vi "PLC_Main.vi"() -> ()   [LabVIEW 2017]
doc: "Andon System cards scanning and ouput ON/OFF through MQTT protocol. Update data in SQL data base for reporting."
uses:
  Control/Andon_demo State.ctl
  <vilib>/addons/database/NI_Database_API.lvlib
  <vilib>/NI/Modbus Library/API/Wrapper/API Main.lvlib
  <vilib>/NI/Modbus Library/API/Wrapper/Create TCP Master.vi
  <vilib>/NI/Modbus Library/API/master/Modbus Master.lvclass
  <vilib>/addons/database/Connection.llb/DB Tools Open Connec (Path).vi
  <vilib>/addons/database/Connection.llb/Conn ObjectReference.ctl
panel:
  out "PLC Status":bool[](array[boolean])
  out "Modbus Instances":refnum<class "Modbus Master.lvclass">[](array[class])
  out "State to Log":T1(array[cluster])
  out "Input Status":bool[][](array[boolean])
  out "Output Status":bool[][](array[boolean])
  in  "stop":bool
  out "Stop from Main":bool
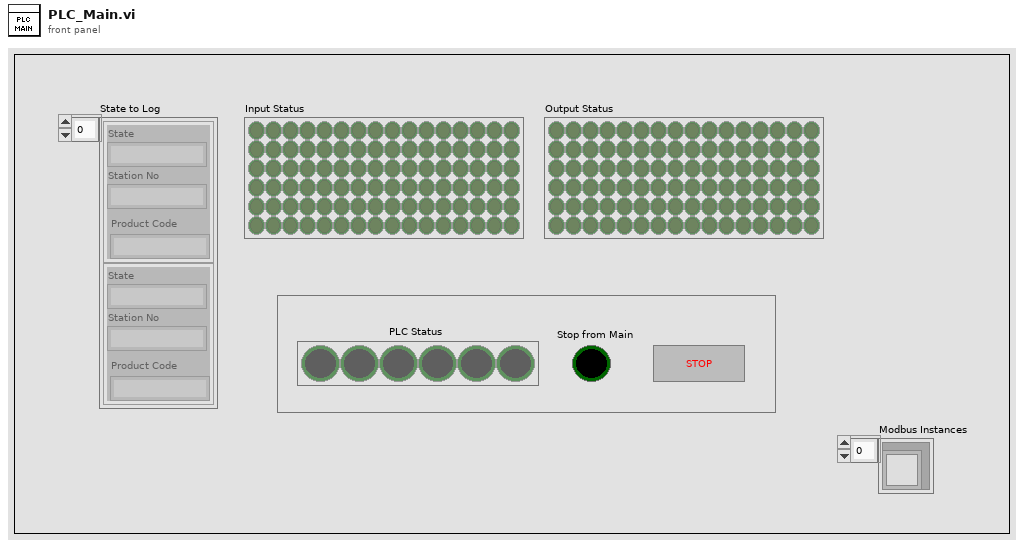
[diagram p1: front panel]
types:
  T1 = cluster{"State":string, "Station No":string, "Product Code":string}[]
  T2 = enum32{"Invalid", "Standard", "Closed", "Hidden", "Minimized", "Maximized"}
  T3 = cluster{"State":string, "Station No":string, "Product Code":string}
  T4 = typedef "Andon_demo State.ctl" = enum16{"Initialise", "Read Inputs", "Process Inputs", "Generate Log Trigger"}
  T5 = cluster{"TCP master instance":refnum<class "Modbus Master.lvclass">, "error out":errorcluster, "CID":string}[]
  T6 = cluster{"TCP master instance":refnum<class "Modbus Master.lvclass">, "error out":errorcluster, "CID":string}
  T7 = cluster{"CID":string, "Comm Stat":bool, "Input":u16[]}
  T8 = typedef "NI_Database_API.lvlib/Conn ObjectReference.ctl" = refnum<k1>
  T9 = cluster{"client name":string, "broker/ server ip address":string[]}
  T10 = cluster{"CID":string, "Comm Stat":bool, "Input":u16[]}[]
  T11 = enum32{"invalid app kind", "Development System", "Run Time System", "Student Edition", "Embedded LabVIEW", "Evaluation", "Custom"}
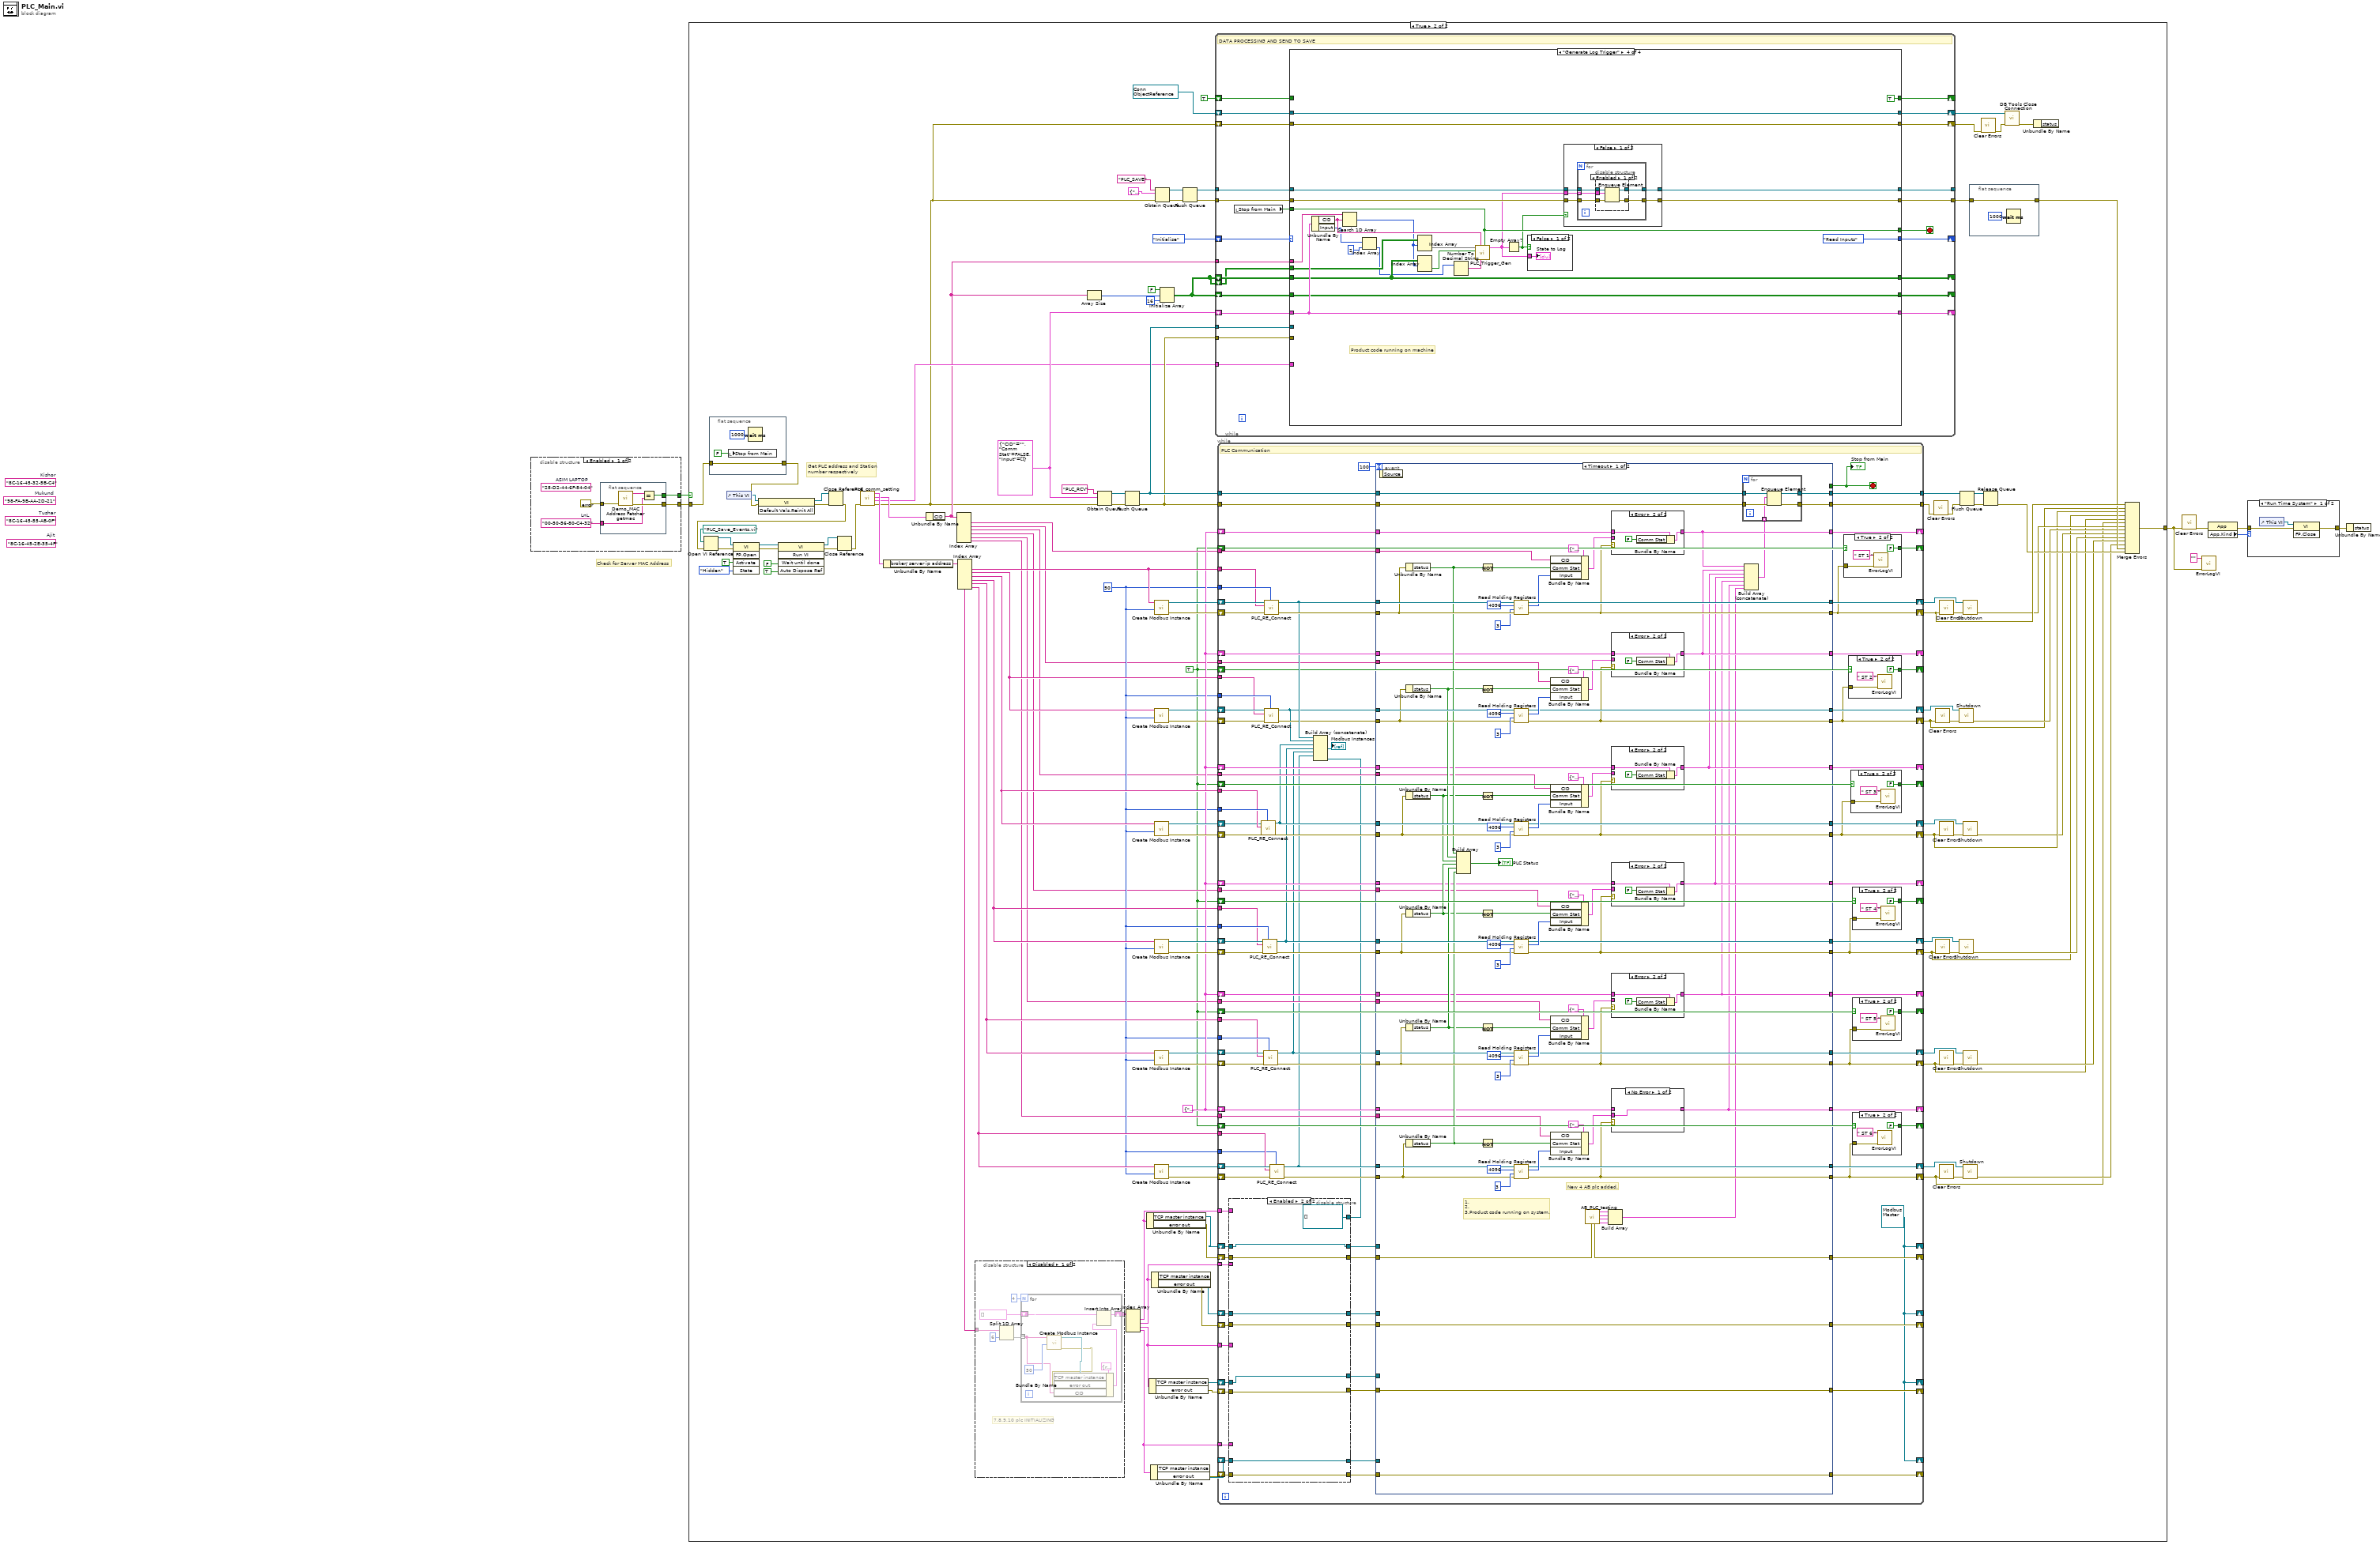
[diagram p0: block diagram]
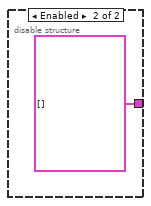
[diagram p3: hidden frame]
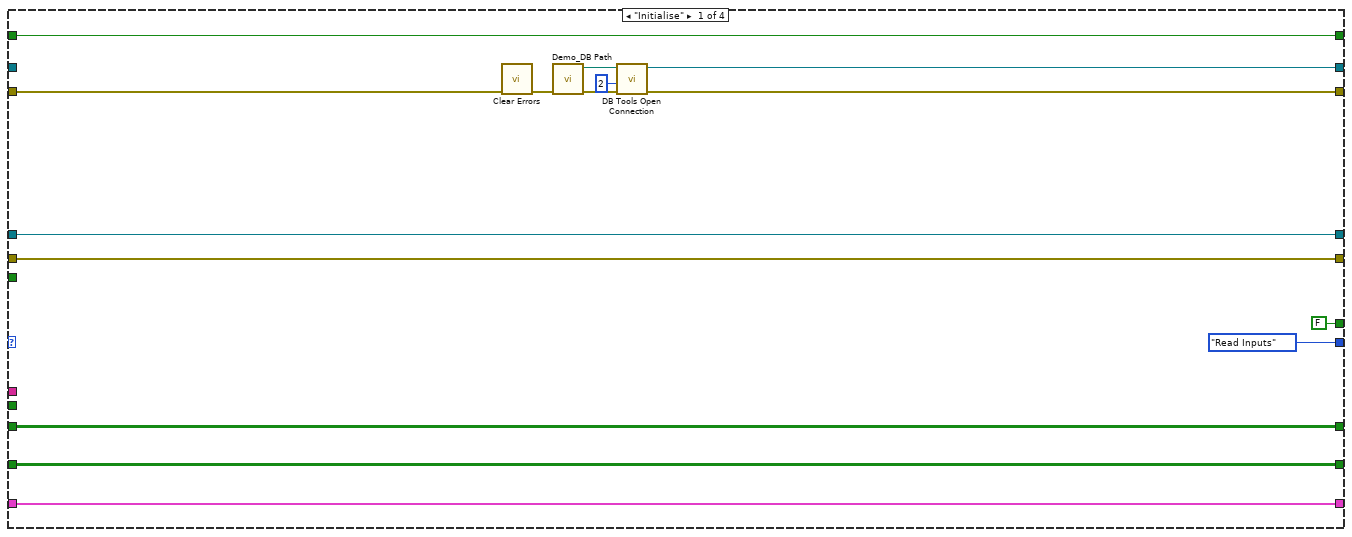
[diagram p4: hidden frame]
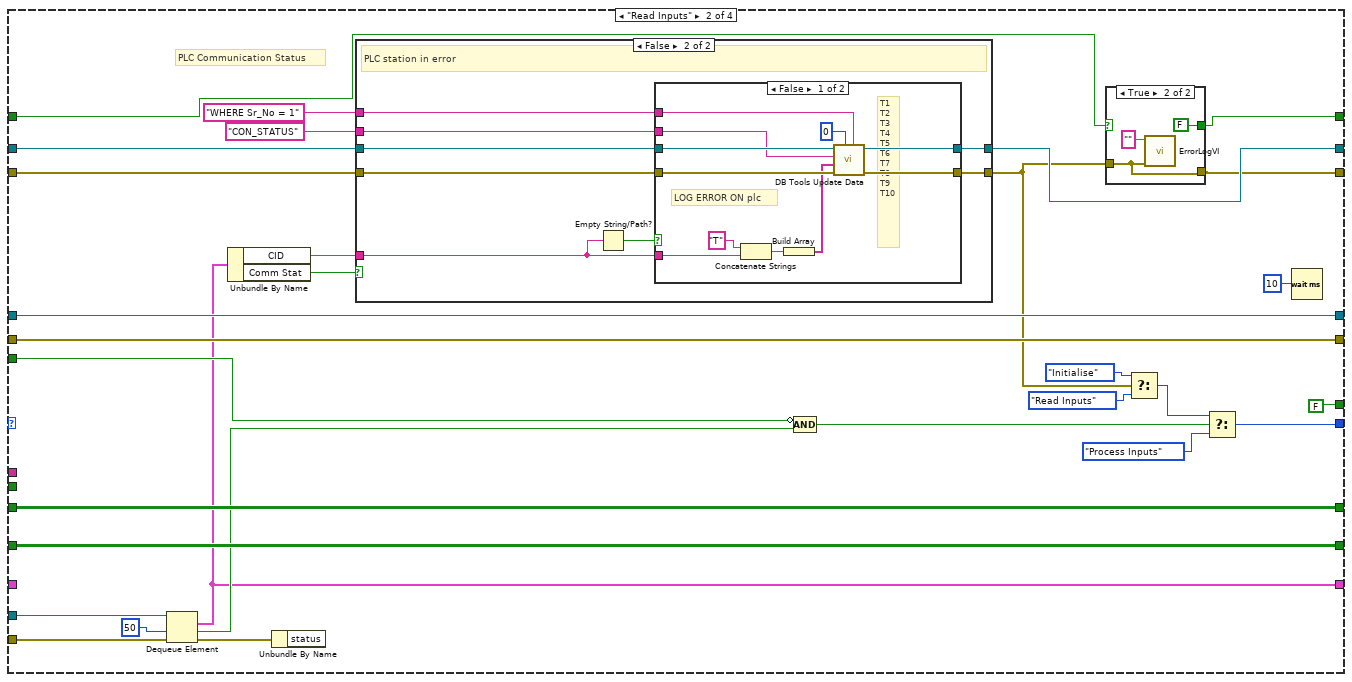
[diagram p5: hidden frame]
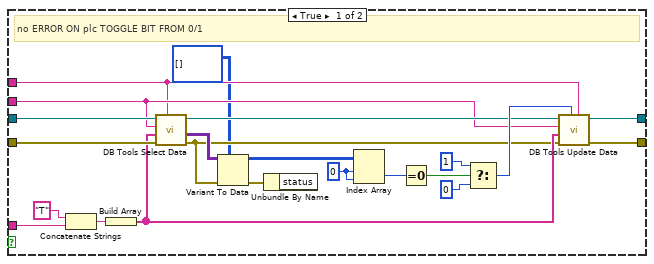
[diagram p7: hidden frame]
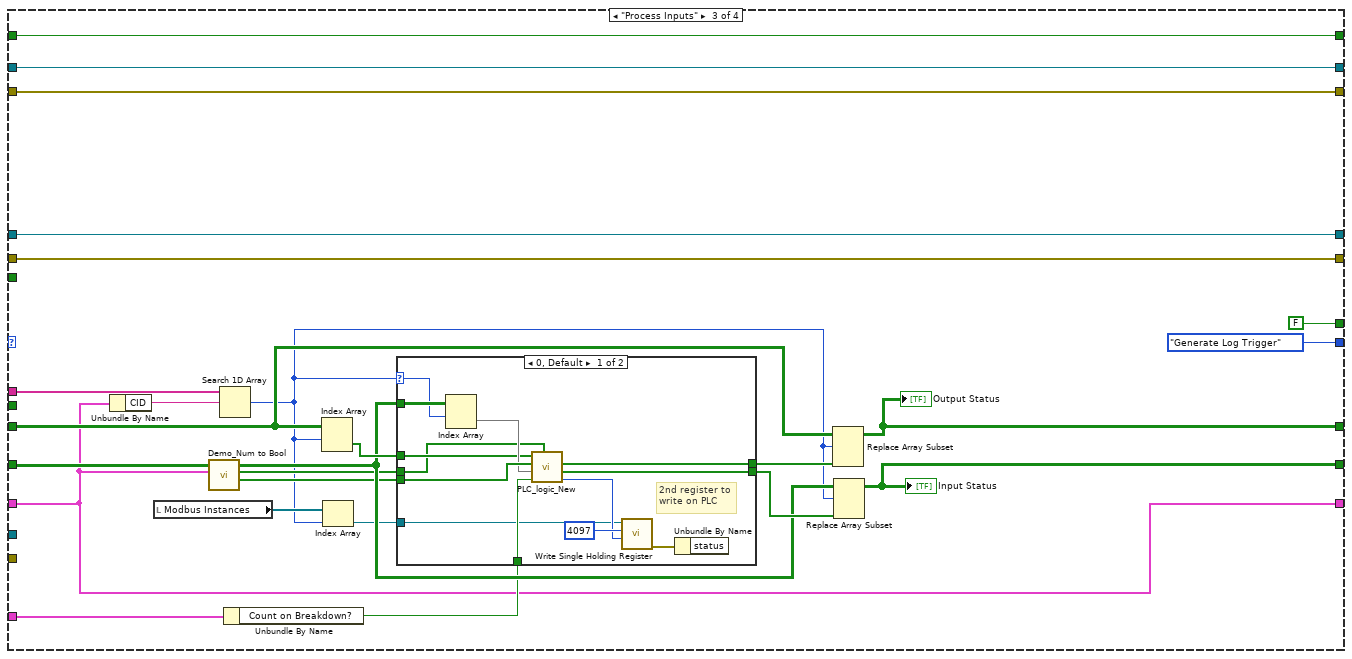
[diagram p9: hidden frame]
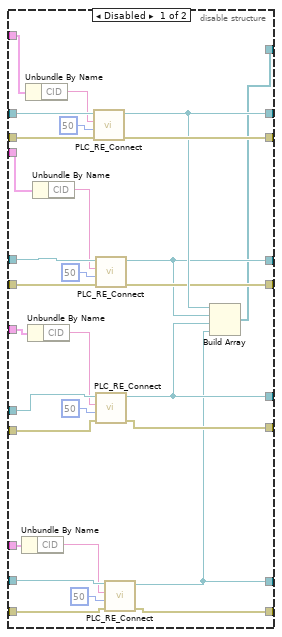
[diagram p14: hidden frame]
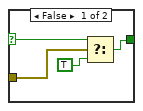
[diagram p15: hidden frame]
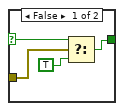
[diagram p16: hidden frame]
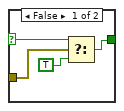
[diagram p17: hidden frame]
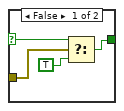
[diagram p18: hidden frame]
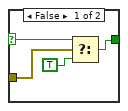
[diagram p19: hidden frame]
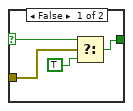
[diagram p20: hidden frame]
diagram:
  (unwired) "8C-16-45-2E-35-4F"  # Ajit
  (unwired) "8C-16-45-55-AB-0F"  # Tushar
  (unwired) "98-FA-9B-AA-2D-21"  # Mukund
  (unwired) "8C-16-45-32-5B-C4"  # Kishor
  # "Check for Server MAC Address"
  n1 = disable-structure shown="Enabled" {
    disable-tunnel: [w11 TRUE] -> w6
    disable-tunnel: [w10 _] -> w2
    frame Enabled {
      (unwired) "28-D2-44-6F-84-04"  # ASIM LAPTOP
      w9 = "00-50-56-80-C4-32"  # LnL
      n2 = flat-sequence {
        tunnel: errorcluster {"status"=FALSE, "code"=0, "source"=""} ("error in (no error)") -> [w17]
        tunnel: [w13] -> w11
        tunnel: [w15] -> w10
        tunnel: w9 -> [w14]
        frame #0 {
          n3 = call "Demo_MAC Address Fetcher getmac.vi"("error in (no error)"=w17) -> ("error out"=w15:errorcluster, "First Matched MAC"=w16:string)  [unwired: 6 in, 3 out]
          n4 = Equal?(x=w16, y=w14) -> (x = y?=w13:bool)
        }
      }
    }
    frame Disabled {
    }
  }
  n5 = case shown="True" w6 {
    tunnel: w2 -> [w19 w48]
    tunnel: [w19 w113] -> w3
    frame False {
    }
    frame True {
      w22 = T8 refnum items=["Connection"] ("connection reference")
      w37 = TRUE
      w82 = T7 {"CID"="", "Comm Stat"=FALSE, "Input"=[]} ("constatnt")
      w83 = T7 {"CID"="", "Comm Stat"=FALSE, "Input"=[]} ("constatnt")
      w68 = 50 ("connect timeout ms")
      # "Get PLC address and Station\nnumber respectively"
      n6 = flat-sequence {
        tunnel: [w156] -> w63
        tunnel: w48 -> [w156]
        frame #0 {
          n7 = local write "Stop from Main"(FALSE ("stop")) -> ()
          n8 = Wait (ms)(milliseconds to wait=u32 1000) -> ()  [unwired: 1 out]
        }
      }
      n9 = control-ref of="This VI"() -> (w62:refnum<vi>)
      n10 = invoke class="VI" method="Default Vals.Reinit All"(reference=w62, error in=w63) -> (reference out=w55:refnum<vi>, error out=w54:errorcluster)  [unwired: 1 in, 1 out]
      n11 = Close Reference(reference=w55, error in (no error)=w54) -> (error out=w64:errorcluster)
      n12 = Open VI Reference(vi path=path "PLC_Save_Events.vi" ("path"), error in (no error)=w64) -> (vi reference=w58:refnum<vi>, error out=w59:errorcluster)  [unwired: 4 in]
      n13 = invoke class="VI" method="FP.Open"(reference=w58, error in=w59, "Activate"=TRUE ("Activate?"), "State"=T2."Hidden") -> (reference out=w56:refnum<vi>, error out=w57:errorcluster)  [unwired: 1 in, 3 out]
      n14 = invoke class="VI" method="Run VI"(reference=w56, error in=w57, "Wait until done"=FALSE ("Wait Until Done"), "Auto Dispose Ref"=TRUE ("Auto Dispose Reference")) -> (reference out=w60:refnum<vi>, error out=w61:errorcluster)  [unwired: 1 in, 3 out]
      n15 = Close Reference(reference=w60, error in (no error)=w61) -> (error out=w47:errorcluster)
      n16 = call "PLC_comm_setting.vi"("error in"=w47) -> ("error out"=w21:errorcluster, "Ignore IsActive"=w46:cluster{"Count on Breakdown?":bool}, "Card Numbers"=w110:cluster{"CID":string[]}, "Comm Setting"=w111:T9)  [unwired: 7 in]
      n17 = Unbundle By Name(w111) -> ("broker/ server ip address"=w36:string[])
      n18 = Unbundle By Name(w110) -> ("CID"=w45:string[])
      n19 = Index Array(array=w45) -> (element #1=w39:string, element #2=w40:string, element #3=w41:string, element #4=w42:string, element #5=w43:string, element #6=w44:string)  [unwired: 6 in]
      n20 = Index Array(array=w36) -> (element #1=w99:string, element #2=w94:string, element #3=w95:string, element #4=w96:string, element #5=w97:string, element #6=w98:string)  [unwired: 6 in]
      n21 = disable-structure shown="Disabled" {
        disable-tunnel: w36 -> [w144 _]
        disable-tunnel: [w141 T5 []] -> w35
        frame Disabled {
          # "7,8,9,10 plc INITIALIZING"
          n22 = Split 1D Array(array=w144, index=6) -> (second subarray=w143:string[])  [unwired: 1 out]
          n23 = for {
            N: 4 -> [_]
            tunnel: w143 -> [w146] mode=indexing
            shift-right: [w152] -> w141
            shift-left: T5 [] -> [w151]
            n24 = call-poly <vilib>:"Create Modbus Instance.vi"("connect timeout ms"=50, "address"=w146) -> ("error out"=w147:errorcluster, "TCP master instance"=w148:refnum<class "Modbus Master.lvclass">)  [unwired: 8 in]
            n25 = Bundle By Name(cluster=T6 {"TCP master instance"=refnum, "error out"={"status"=FALSE, "code"=0, "source"=""}, "CID"=""} ("Cluster"), "TCP master instance"=w148, "error out"=w147, "CID"=w146) -> (w150:T6)
            n26 = Insert Into Array(array=w151, new element=w150) -> (w152:T5)  [unwired: 1 in]
          }
        }
        frame Enabled {
        }
      }
      n27 = Array Size(array=w45) -> (size(s)=w121:i32)
      n28 = Obtain Queue(name (unnamed)="PLC_RCV", element data type=w83, error in (no error)=w21) -> (queue out=w135:refnum<queue>, error out=w133:errorcluster)  [unwired: 2 in, 1 out]
      n29 = Flush Queue(queue=w135, error in (no error)=w133) -> (queue out=w134:refnum<queue>, error out=w124:errorcluster)  [unwired: 1 out]
      n30 = Index Array(array=w35) -> (element #1=w32:T6, element #2=w29:T6, element #3=w23:T6, element #4=w26:T6)  [unwired: 4 in]
      n31 = Unbundle By Name(w32) -> ("TCP master instance"=w34:refnum<class "Modbus Master.lvclass">, "error out"=w33:errorcluster)
      n32 = Unbundle By Name(w23) -> ("TCP master instance"=w24:refnum<class "Modbus Master.lvclass">, "error out"=w25:errorcluster)
      n33 = Unbundle By Name(w26) -> ("TCP master instance"=w28:refnum<class "Modbus Master.lvclass">, "error out"=w27:errorcluster)
      n34 = Unbundle By Name(w29) -> ("TCP master instance"=w31:refnum<class "Modbus Master.lvclass">, "error out"=w30:errorcluster)
      n35 = call-poly <vilib>:"Create Modbus Instance.vi"("connect timeout ms"=w68, "address"=w99) -> ("error out"=w119:errorcluster, "TCP master instance"=w118:refnum<class "Modbus Master.lvclass">)  [unwired: 8 in]
      n36 = call-poly <vilib>:"Create Modbus Instance.vi"("connect timeout ms"=w68, "address"=w94) -> ("error out"=w108:errorcluster, "TCP master instance"=w109:refnum<class "Modbus Master.lvclass">)  [unwired: 8 in]
      n37 = call-poly <vilib>:"Create Modbus Instance.vi"("connect timeout ms"=w68, "address"=w95) -> ("error out"=w107:errorcluster, "TCP master instance"=w106:refnum<class "Modbus Master.lvclass">)  [unwired: 8 in]
      n38 = call-poly <vilib>:"Create Modbus Instance.vi"("connect timeout ms"=w68, "address"=w96) -> ("error out"=w103:errorcluster, "TCP master instance"=w102:refnum<class "Modbus Master.lvclass">)  [unwired: 8 in]
      n39 = call-poly <vilib>:"Create Modbus Instance.vi"("connect timeout ms"=w68, "address"=w97) -> ("error out"=w104:errorcluster, "TCP master instance"=w105:refnum<class "Modbus Master.lvclass">)  [unwired: 8 in]
      n40 = call-poly <vilib>:"Create Modbus Instance.vi"("connect timeout ms"=w68, "address"=w98) -> ("error out"=w101:errorcluster, "TCP master instance"=w100:refnum<class "Modbus Master.lvclass">)  [unwired: 8 in]
      n41 = Obtain Queue(name (unnamed)="PLC_SAVE", element data type=T3 {"State"="MAINT_Trigger", "Station No"="", "Product Code"=""} ("States to Log"), error in (no error)=w21) -> (queue out=w128:refnum<queue>, error out=w127:errorcluster)  [unwired: 2 in, 1 out]
      n42 = Initialize Array(FALSE, w121, 16 ("dimension size")) -> (w122:bool[][])
      n43 = Flush Queue(queue=w128, error in (no error)=w127) -> (queue out=w126:refnum<queue>, error out=w125:errorcluster)  [unwired: 1 out]
      n44 = while {
        tunnel: w134 -> [w183]
        shift-right: [w182] -> _
        shift-left: w83 -> [w181]
        shift-right: [w180] -> _
        shift-left: Andon_demo_State."Initialise" -> [w184]
        shift-right: [w178] -> _
        shift-left: w122 -> [w179]
        shift-right: [w176] -> _
        shift-left: w122 -> [w177]
        tunnel: w45 -> [w175]
        tunnel: w126 -> [w174]
        tunnel: w125 -> [w173]
        tunnel: [w172] -> _
        tunnel: [w171] -> w123
        tunnel: w124 -> [w168]
        shift-left: w122 -> [w167]
        tunnel: w46 -> [w166]
        shift-right: [w164] -> w67
        shift-left: w22 -> [w165]
        shift-right: [w163] -> w66
        shift-left: w21 -> [w162]
        shift-right: [w160] -> _
        shift-left: TRUE -> [w161]
        stop <- w170 stop-if-true
        # "DATA PROCESSING AND SEND TO SAVE"
        n45 = local read "Stop from Main"() -> (w169:bool)
        n46 = case shown="\"Generate Log Trigger\"" w184 {
          tunnel: w183 -> [_ w229 _ _]
          tunnel: [w194 w211 w285 w338] -> w182
          tunnel: w181 -> [w194 _ w285 w338]
          tunnel: [Andon_demo_State."Read Inputs" w221 Andon_demo_State."Generate Log Trigger" Andon_demo_State."Read Inputs"] -> w180
          tunnel: w179 -> [w196 w227 w296 w325]
          tunnel: [w196 w227 w300 w325] -> w178
          tunnel: w177 -> [w195 w226 w289 w336]
          tunnel: [w195 w226 w298 w336] -> w176
          tunnel: w175 -> [_ _ w297 w340]
          tunnel: w167 -> [_ _ _ w337]
          tunnel: w174 -> [w199 w225 w295 w335]
          tunnel: w173 -> [w198 w224 w294 w334]
          tunnel: [w199 w225 w295 w333] -> w172
          tunnel: [w198 w224 w294 w332] -> w171
          tunnel: [FALSE ("Stop from Main") FALSE ("STOP FROM MAIN") FALSE ("STOP FROM MAIN") w331] -> w170
          tunnel: w169 -> [_ w220 _ w331]
          tunnel: w168 -> [_ w218 _ _]
          tunnel: w166 -> [_ _ w288 _]
          tunnel: w165 -> [_ w215 w286 w330]
          tunnel: w162 -> [w190 w214 w279 w322]
          tunnel: [w188 w213 w286 w330] -> w164
          tunnel: [w187 w200 w279 w322] -> w163
          tunnel: w161 -> [w185 w203 w278 _]
          tunnel: [w185 w202 w278 TRUE] -> w160
          frame "Initialise" {
            n47 = call <vilib>:"Clear Errors.vi"("error in (no error)"=w190) -> ("error out"=w189:errorcluster)  [unwired: 5 in, 1 out]
            n48 = call "Demo_DB Path.vi"("error in"=w189) -> ("error out"=w192:errorcluster, "DB Path"=w193:path)  [unwired: 9 in]
            n49 = call-poly <vilib>:"DB Tools Open Connection.vi"("error in (no error)"=w192, "connection timeout (15)"=2, "connection information"=w193) -> ("error out"=w187:errorcluster, "connection reference"=w188:T8)  [unwired: 5 in]
          }
          frame "Read Inputs" {
            # "PLC Communication Status"
            n50 = Dequeue Element(queue=w229, timeout in ms (-1)=50, error in (no error)=w218) -> (element=w211:T7, timed out?=w216:bool, error out=w212:errorcluster)  [unwired: 1 out]
            n51 = Unbundle By Name(w211) -> ("CID"=w210:string, "Comm Stat"=w209:bool)
            n52 = Unbundle By Name(w212) -> ()  [unwired: 1 out]
            n53 = case shown="False" w209 {
              tunnel: w215 -> [w248 w264]
              tunnel: w214 -> [w246 w263]
              tunnel: [w256 w262] -> w213
              tunnel: w210 -> [w255 w261]
              tunnel: [w249 w260] -> w201
              tunnel: "WHERE Sr_No = 1" ("condition") -> [w243 w258]
              tunnel: "CON_STATUS" ("table") -> [w245 w257]
              frame True {
                w237 = 0 ("disabled index (col)")
                # "no ERROR ON plc TOGGLE BIT FROM 0/1"
                n54 = Concatenate Strings("T" ("string"), w255) -> (w251:string)
                n55 = Build Array(w251) -> (w244:string[])
                n56 = call <vilib>:"DB Tools Select Data.vi"("condition"=w243, "error in (no error)"=w246, "columns"=w244, "table"=w245, "connection reference"=w248) -> ("error out"=w241:errorcluster, "data"=w242:variant[][], "connection reference out"=w247:T8)  [unwired: 1 in]
                n57 = Variant To Data(error in=w241, type=i32[][] [], Variant=w242) -> (data=w238:i32[][], error out=w240:errorcluster)
                n58 = Unbundle By Name(w240) -> ()  [unwired: 1 out]
                n59 = Index Array(array=w238, index (row)=w237, index (col)=w237) -> (element=w236:i32)
                n60 = Equal To 0?(x=w236) -> (x = 0?=w235:bool)
                n61 = Select(t=1, s=w235, f=0) -> (s? t:f=w252:i32)
                n62 = call <vilib>:"DB Tools Update Data.vi"("condition"=w243, "data"=w252, "error in (no error)"=w241, "columns"=w244, "table"=w245, "connection reference"=w247) -> ("error out"=w249:errorcluster, "connection reference out"=w256:T8)  [unwired: 4 in]
              }
              frame False {
                # "PLC station in error"
                n63 = Empty String/Path?(string/path=w261) -> (empty?=w259:bool)
                n64 = case shown="False" w259 {
                  tunnel: w264 -> [w275 w277]
                  tunnel: w263 -> [w274 w276]
                  tunnel: [w273 w277] -> w262
                  tunnel: w261 -> [w268 _]
                  tunnel: [w267 w276] -> w260
                  tunnel: w258 -> [w266 _]
                  tunnel: w257 -> [w265 _]
                  frame False {
                    # "LOG ERROR ON plc"
                    # "T1\nT2\nT3\nT4\nT5\nT6\nT7\nT8\nT9\nT10"
                    n65 = Concatenate Strings("T" ("string"), w268) -> (w271:string)
                    n66 = Build Array(w271) -> (w272:string[])
                    n67 = call <vilib>:"DB Tools Update Data.vi"("condition"=w266, "data"=0, "error in (no error)"=w274, "columns"=w272, "table"=w265, "connection reference"=w275) -> ("error out"=w267:errorcluster, "connection reference out"=w273:T8)  [unwired: 4 in]
                  }
                  frame True {
                  }
                }
              }
            }
            n68 = Compound Arithmetic op=AND(invert w220, w216) -> (w219:bool)
            n69 = case shown="True" w203 {
              selector: w203 -> [w231 _]
              tunnel: w201 -> [w230 w232]
              tunnel: [w231 FALSE] -> w202
              tunnel: [w230 w232] -> w200
              frame False {
              }
              frame True {
                n70 = call "ErrorLogVI.vi"("Error In"=w232, "Station"="") -> ()  [unwired: 10 in]
              }
            }
            n71 = Select(t=Andon_demo_State."Initialise", s=w201, f=Andon_demo_State."Read Inputs") -> (s? t:f=w206:T4)
            n72 = Select(t=w206, s=w219, f=Andon_demo_State."Process Inputs") -> (s? t:f=w221:T4)
            n73 = Wait (ms)(milliseconds to wait=u32 10) -> ()  [unwired: 1 out]
          }
          frame "Process Inputs" {
            n74 = Unbundle By Name(w285) -> ("CID"=w290:string)
            n75 = local read "Modbus Instances"() -> (w282:refnum<class "Modbus Master.lvclass">[])
            n76 = call "Demo_Num to Bool.vi"("PLC_Data"=w285) -> ("Input Array"=w284:bool[], "Output Array"=w283:bool[])  [unwired: 8 in, 1 out]
            n77 = Search 1D Array(1D array=w297, element=w290) -> (index of element=w281:i32)  [unwired: 1 in]
            n78 = Unbundle By Name(w288) -> ("Count on Breakdown?"=w287:bool)
            n79 = Index Array(array=w296, index (row)=w281) -> (element=w291:bool[])  [unwired: 1 in]
            n80 = Index Array(array=w282, index=w281) -> (element=w280:refnum<class "Modbus Master.lvclass">)
            n81 = case shown="0, Default" w281 {
              selector: w281 -> [w306 _]
              tunnel: w284 -> [w312 w315]
              tunnel: [w307 w315] -> w299
              tunnel: [w308 w316] -> w292
              tunnel: w291 -> [w310 w316]
              tunnel: w289 -> [w313 _]
              tunnel: w287 -> [w314 _]
              tunnel: w283 -> [w309 _]
              tunnel: w280 -> [w302 _]
              frame 0, Default {
                # "2nd register to\nwrite on PLC"
                n82 = Index Array(array=w313, index (row)=w306) -> (element=w311:bool[])  [unwired: 1 in]
                n83 = call "PLC_logic_New.vi"("Trigger"=w309, "IsActive?"=w314, "Inputs past"=w311, "Inputs"=w312, "Outputs past"=w310) -> ("Output Data"=w303:u16, "Inputs to save"=w307:bool[], "Outputs OUT"=w308:bool[])  [unwired: 3 in, 1 out]
                n84 = call-dynamic "Write Single Holding Register.vi"("register to write"=w303, "address"=u16 4097 ("starting address"), "Modbus master in"=w302) -> ("error out"=w305:errorcluster)  [unwired: 7 in, 1 out]
                n85 = Unbundle By Name(w305) -> ()  [unwired: 1 out]
              }
              frame -1 {
              }
            }
            n86 = Replace Array Subset(array=w296, new element=w292, index (row)=w281) -> (w300:bool[][])  [unwired: 1 in]
            "Output Status" <- w300
            n87 = Replace Array Subset(array=w289, new element=w299, index (row)=w281) -> (w298:bool[][])  [unwired: 1 in]
            "Input Status" <- w298
          }
          frame "Generate Log Trigger" {
            # "Product code running on machine"
            n88 = Unbundle By Name(w338) -> ("CID"=w326:string, "Input"=w320:u16[])
            n89 = Search 1D Array(1D array=w340, element=w326) -> (index of element=w324:i32)  [unwired: 1 in]
            n90 = Index Array(array=w320, index=2) -> (element=w318:u16)
            n91 = Index Array(array=w337, index (row)=w324) -> (element=w328:bool[])  [unwired: 1 in]
            n92 = Index Array(array=w325, index (row)=w324) -> (element=w327:bool[])  [unwired: 1 in]
            n93 = Number To Decimal String(number=w318) -> (decimal integer string=w317:string)  [unwired: 1 in]
            n94 = call "PLC_Trigger_Gen.vi"("0_Stop"=w331, "Product Code"=w317, "Station Number"=w326, "Trig"=w327, "Trig old"=w328) -> ("State to Log"=w329:T1)  [unwired: 6 in]
            n95 = Empty Array?(array=w329) -> (empty?=w323:bool)
            n96 = case shown="False" w323 {
              tunnel: w329 -> [w360 _]
              frame False {
                "State to Log" <- w360
              }
              frame True {
              }
            }
            n97 = case shown="False" w323 {
              tunnel: w335 -> [w345 w359]
              tunnel: w334 -> [w344 w358]
              tunnel: [w343 w359] -> w333
              tunnel: [w342 w358] -> w332
              tunnel: w329 -> [w341 _]
              frame False {
                n98 = for {
                  tunnel: w344 -> [w349]
                  tunnel: [w347] -> w342
                  tunnel: w345 -> [w350]
                  tunnel: [w348] -> w343
                  tunnel: w341 -> [w346] mode=indexing
                  n99 = disable-structure shown="Enabled" {
                    disable-tunnel: w350 -> [w355 w357]
                    disable-tunnel: w349 -> [w354 w356]
                    disable-tunnel: [w353 w357] -> w348
                    disable-tunnel: [w352 w356] -> w347
                    disable-tunnel: w346 -> [w351 _]
                    frame Enabled {
                      n100 = Enqueue Element(queue=w355, element=w351, error in (no error)=w354) -> (queue out=w353:refnum<queue>, error out=w352:errorcluster)  [unwired: 1 in, 1 out]
                    }
                    frame Disabled {
                    }
                  }
                }
              }
              frame True {
              }
            }
          }
        }
      }
      n101 = while {
        tunnel: w124 -> [w471]
        tunnel: [w470] -> w115
        tunnel: w134 -> [w469]
        tunnel: [w468] -> w136
        shift-right: [w422] -> w112
        shift-left: w119 -> [w465]
        tunnel: w68 -> [w463]
        tunnel: w99 -> [w462]
        shift-right: [w460] -> w116
        shift-left: w118 -> [w464]
        shift-right: [w433] -> w77
        shift-left: w108 -> [w416]
        tunnel: w68 -> [w412]
        tunnel: w94 -> [w411]
        shift-right: [w459] -> w84
        shift-left: w109 -> [w414]
        shift-right: [w428] -> w76
        shift-left: w107 -> [w409]
        tunnel: w68 -> [w408]
        tunnel: w95 -> [w407]
        shift-right: [w458] -> w85
        shift-left: w106 -> [w406]
        shift-right: [w429] -> w69
        shift-left: w103 -> [w402]
        tunnel: w68 -> [w400]
        tunnel: w96 -> [w399]
        shift-right: [w457] -> w86
        shift-left: w102 -> [w401]
        shift-right: [w426] -> w70
        shift-left: w104 -> [w397]
        tunnel: w68 -> [w395]
        tunnel: w97 -> [w394]
        shift-right: [w456] -> w87
        shift-left: w105 -> [w396]
        shift-right: [w424] -> w71
        shift-left: w101 -> [w391]
        tunnel: w68 -> [w387]
        tunnel: w98 -> [w388]
        shift-right: [w455] -> w88
        shift-left: w100 -> [w389]
        shift-right: [w451] -> _
        shift-left: w82 -> [w443]
        shift-right: [w450] -> _
        shift-left: w82 -> [w444]
        shift-right: [w449] -> _
        shift-left: w82 -> [w445]
        shift-right: [w448] -> _
        shift-left: w82 -> [w446]
        shift-right: [w452] -> _
        shift-left: w82 -> [w447]
        shift-right: [w454] -> _
        shift-left: w82 -> [w453]
        tunnel: w44 -> [w435]
        tunnel: w43 -> [w436]
        tunnel: w42 -> [w437]
        tunnel: w41 -> [w438]
        tunnel: w40 -> [w439]
        tunnel: w39 -> [w440]
        shift-right: [w434] -> _
        shift-left: w37 -> [w432]
        shift-right: [w431] -> _
        shift-left: w37 -> [w418]
        shift-right: [w430] -> _
        shift-left: w37 -> [w419]
        shift-right: [w427] -> _
        shift-left: w37 -> [w420]
        shift-right: [w425] -> _
        shift-left: w37 -> [w421]
        shift-right: [w423] -> _
        shift-left: w37 -> [w417]
        shift-right: [w361] -> _
        shift-left: w31 -> [w380]
        shift-right: [w361] -> _
        shift-left: w34 -> [w385]
        shift-right: [w361] -> _
        shift-left: w28 -> [w377]
        shift-right: [w361] -> _
        shift-left: w24 -> [w376]
        shift-right: [w369] -> _
        shift-left: w33 -> [w386]
        shift-right: [w368] -> _
        shift-left: w30 -> [w381]
        shift-right: [w367] -> _
        shift-left: w25 -> [w375]
        shift-right: [w366] -> _
        shift-left: w27 -> [w378]
        tunnel: w32 -> [w365]
        tunnel: w29 -> [w364]
        tunnel: w26 -> [w363]
        tunnel: w23 -> [w362]
        stop <- w467 stop-if-true
        w361 = refnum<class "Modbus Master.lvclass"> refnum ("TCP master instance")
        # "PLC Communication"
        n102 = disable-structure shown="Enabled" {
          disable-tunnel: w386 -> [w500 w506]
          disable-tunnel: w385 -> [w499 w507]
          disable-tunnel: [w497 w506] -> w384
          disable-tunnel: [w496 w507] -> w383
          disable-tunnel: [w494 w509] -> w382
          disable-tunnel: w381 -> [w493 w509]
          disable-tunnel: w380 -> [w492 w508]
          disable-tunnel: [w491 w508] -> w379
          disable-tunnel: w378 -> [w488 w502]
          disable-tunnel: w377 -> [w487 w503]
          disable-tunnel: w376 -> [w486 w505]
          disable-tunnel: w375 -> [w485 w504]
          disable-tunnel: [w484 w504] -> w374
          disable-tunnel: [w483 w502] -> w373
          disable-tunnel: [w482 w505] -> w372
          disable-tunnel: [w481 w503] -> w371
          disable-tunnel: [w480 refnum<class "Modbus Master.lvclass">[] []] -> w370
          disable-tunnel: w365 -> [w479 _]
          disable-tunnel: w364 -> [w477 _]
          disable-tunnel: w363 -> [w474 _]
          disable-tunnel: w362 -> [w473 _]
          frame Disabled {
            n103 = Unbundle By Name(w474) -> ("CID"=w475:string)
            n104 = Unbundle By Name(w479) -> ("CID"=w478:string)
            n105 = Unbundle By Name(w473) -> ("CID"=w472:string)
            n106 = Unbundle By Name(w477) -> ("CID"=w476:string)
            n107 = call "PLC_RE_Connect.vi"("error in (no error)"=w500, "port (502)"=50 ("connect timeout ms"), "CID"=w478, "Modbus Master in"=w499) -> ("error out"=w497:errorcluster, "Modbus Master out"=w496:refnum<class "Modbus Master.lvclass">)  [unwired: 6 in]
            n108 = call "PLC_RE_Connect.vi"("error in (no error)"=w493, "port (502)"=50 ("connect timeout ms"), "CID"=w476, "Modbus Master in"=w492) -> ("error out"=w494:errorcluster, "Modbus Master out"=w491:refnum<class "Modbus Master.lvclass">)  [unwired: 6 in]
            n109 = call "PLC_RE_Connect.vi"("error in (no error)"=w485, "port (502)"=50 ("connect timeout ms"), "CID"=w472, "Modbus Master in"=w486) -> ("error out"=w484:errorcluster, "Modbus Master out"=w482:refnum<class "Modbus Master.lvclass">)  [unwired: 6 in]
            n110 = call "PLC_RE_Connect.vi"("error in (no error)"=w488, "port (502)"=50 ("connect timeout ms"), "CID"=w475, "Modbus Master in"=w487) -> ("error out"=w483:errorcluster, "Modbus Master out"=w481:refnum<class "Modbus Master.lvclass">)  [unwired: 6 in]
            n111 = Build Array(w496, w491, w482, w481) -> (w480:refnum<class "Modbus Master.lvclass">[])
          }
          frame Enabled {
          }
        }
        n112 = call "PLC_RE_Connect.vi"("connect timeout ms"=w408, "error in (no error)"=w409, "CID"=w407, "Modbus Master in"=w406) -> ("error out"=w410:errorcluster, "Modbus Master out"=w405:refnum<class "Modbus Master.lvclass">)  [unwired: 6 in]
        n113 = call "PLC_RE_Connect.vi"("connect timeout ms"=w400, "error in (no error)"=w402, "CID"=w399, "Modbus Master in"=w401) -> ("error out"=w403:errorcluster, "Modbus Master out"=w404:refnum<class "Modbus Master.lvclass">)  [unwired: 6 in]
        n114 = call "PLC_RE_Connect.vi"("connect timeout ms"=w395, "error in (no error)"=w397, "CID"=w394, "Modbus Master in"=w396) -> ("error out"=w398:errorcluster, "Modbus Master out"=w393:refnum<class "Modbus Master.lvclass">)  [unwired: 6 in]
        n115 = call "PLC_RE_Connect.vi"("connect timeout ms"=w463, "error in (no error)"=w465, "CID"=w462, "Modbus Master in"=w464) -> ("error out"=w461:errorcluster, "Modbus Master out"=w442:refnum<class "Modbus Master.lvclass">)  [unwired: 6 in]
        n116 = call "PLC_RE_Connect.vi"("connect timeout ms"=w412, "error in (no error)"=w416, "CID"=w411, "Modbus Master in"=w414) -> ("error out"=w415:errorcluster, "Modbus Master out"=w413:refnum<class "Modbus Master.lvclass">)  [unwired: 6 in]
        n117 = call "PLC_RE_Connect.vi"("connect timeout ms"=w387, "error in (no error)"=w391, "CID"=w388, "Modbus Master in"=w389) -> ("error out"=w392:errorcluster, "Modbus Master out"=w390:refnum<class "Modbus Master.lvclass">)  [unwired: 6 in]
        n118 = Build Array (concatenate)(w442, w413, w405, w404, w393, w390, w370) -> (→"Modbus Instances":refnum<class "Modbus Master.lvclass">[])
        n119 = event shown="[0] Timeout" {
          selector: _ -> [_ _]
          dyn-events: _ -> [_ _]
          timeout: 100 -> [_ _]
          tunnel: [_ w683] -> w467
          tunnel: [w646 w702] -> w470
          tunnel: w471 -> [w647 w702]
          tunnel: [w648 w701] -> w468
          tunnel: w469 -> [w649 w701]
          tunnel: w442 -> [w651 w700]
          tunnel: w461 -> [w645 w682]
          tunnel: [w650 w700] -> w460
          tunnel: [w598 w681] -> w422
          tunnel: [w603 w699] -> w459
          tunnel: w413 -> [w604 w699]
          tunnel: [w585 w698] -> w433
          tunnel: w415 -> [w602 w698]
          tunnel: [w605 w697] -> w458
          tunnel: w405 -> [w606 w697]
          tunnel: w410 -> [w601 w696]
          tunnel: [w580 w696] -> w428
          tunnel: [w607 w695] -> w457
          tunnel: w404 -> [w608 w695]
          tunnel: [w577 w694] -> w429
          tunnel: w403 -> [w600 w694]
          tunnel: [w610 w693] -> w456
          tunnel: w393 -> [w611 w693]
          tunnel: [w575 w692] -> w426
          tunnel: w398 -> [w609 w692]
          tunnel: [w613 w691] -> w455
          tunnel: w390 -> [w614 w691]
          tunnel: [w571 w690] -> w424
          tunnel: w392 -> [w612 w690]
          tunnel: [w568 w684] -> w454
          tunnel: w453 -> [w569 w684]
          tunnel: [w572 w685] -> w452
          tunnel: [w596 w688] -> w451
          tunnel: [w584 w689] -> w450
          tunnel: [w581 w687] -> w449
          tunnel: [w576 w686] -> w448
          tunnel: w447 -> [w573 w685]
          tunnel: w446 -> [w578 w686]
          tunnel: w445 -> [w582 w687]
          tunnel: w444 -> [w586 w689]
          tunnel: w443 -> [w597 w688]
          tunnel: w440 -> [w567 _]
          tunnel: w439 -> [w566 _]
          tunnel: w438 -> [w565 _]
          tunnel: w437 -> [w564 _]
          tunnel: w436 -> [w563 _]
          tunnel: w435 -> [w562 _]
          tunnel: w384 -> [w558 _]
          tunnel: w383 -> [_ _]
          tunnel: w379 -> [_ _]
          tunnel: w382 -> [w561 _]
          tunnel: w374 -> [w560 _]
          tunnel: w373 -> [w559 _]
          tunnel: w371 -> [_ _]
          tunnel: w372 -> [_ _]
          tunnel: [w557 _] -> w369
          tunnel: [w561 _] -> w368
          tunnel: [w560 _] -> w367
          tunnel: [w559 _] -> w366
          event Timeout {
            # "New 4 AB plc added."
            # "1.\n2.\n3.Product code running on system."
            n120 = event-data() -> ()  [unwired: 1 in, 1 out]
            n121 = Unbundle By Name(w645) -> ("status"=w594:bool)
            n122 = Unbundle By Name(w602) -> ("status"=w590:bool)
            n123 = Unbundle By Name(w601) -> ("status"=w589:bool)
            n124 = Unbundle By Name(w600) -> ("status"=w591:bool)
            n125 = Unbundle By Name(w609) -> ("status"=w592:bool)
            n126 = Unbundle By Name(w612) -> ("status"=w593:bool)
            n127 = Build Array(w594, w590, w589, w591, w592, w593) -> (→"PLC Status":bool[])
            n128 = Not(x=w594) -> (.not. x?=w644:bool)
            n129 = Not(x=w590) -> (.not. x?=w635:bool)
            n130 = Not(x=w589) -> (.not. x?=w634:bool)
            n131 = Not(x=w591) -> (.not. x?=w625:bool)
            n132 = Not(x=w592) -> (.not. x?=w624:bool)
            n133 = Not(x=w593) -> (.not. x?=w615:bool)
            n134 = call-dynamic "Read Holding Registers.vi"("error in"=w645, "number of inputs"=u16 3, "starting address"=u16 4096, "Modbus master in"=w651) -> ("error out"=w598:errorcluster, "register values"=w643:u16[], "Modbus master out"=w650:refnum<class "Modbus Master.lvclass">)  [unwired: 5 in]
            n135 = call-dynamic "Read Holding Registers.vi"("error in"=w602, "number of inputs"=u16 3, "starting address"=u16 4096, "Modbus master in"=w604) -> ("error out"=w585:errorcluster, "register values"=w636:u16[], "Modbus master out"=w603:refnum<class "Modbus Master.lvclass">)  [unwired: 5 in]
            n136 = call-dynamic "Read Holding Registers.vi"("error in"=w601, "number of inputs"=u16 3, "starting address"=u16 4096, "Modbus master in"=w606) -> ("error out"=w580:errorcluster, "register values"=w633:u16[], "Modbus master out"=w605:refnum<class "Modbus Master.lvclass">)  [unwired: 5 in]
            n137 = call-dynamic "Read Holding Registers.vi"("error in"=w600, "number of inputs"=u16 3, "starting address"=u16 4096, "Modbus master in"=w608) -> ("error out"=w577:errorcluster, "register values"=w626:u16[], "Modbus master out"=w607:refnum<class "Modbus Master.lvclass">)  [unwired: 5 in]
            n138 = call-dynamic "Read Holding Registers.vi"("error in"=w609, "number of inputs"=u16 3, "starting address"=u16 4096, "Modbus master in"=w611) -> ("error out"=w575:errorcluster, "register values"=w623:u16[], "Modbus master out"=w610:refnum<class "Modbus Master.lvclass">)  [unwired: 5 in]
            n139 = call-dynamic "Read Holding Registers.vi"("error in"=w612, "number of inputs"=u16 3, "starting address"=u16 4096, "Modbus master in"=w614) -> ("error out"=w571:errorcluster, "register values"=w616:u16[], "Modbus master out"=w613:refnum<class "Modbus Master.lvclass">)  [unwired: 5 in]
            n140 = Bundle By Name(cluster=T7 {"CID"="", "Comm Stat"=FALSE, "Input"=[]} ("constatnt"), "CID"=w567, "Comm Stat"=w644, "Input"=w643) -> (w599:T7)
            n141 = Bundle By Name(cluster=T7 {"CID"="", "Comm Stat"=FALSE, "Input"=[]} ("constatnt"), "CID"=w566, "Comm Stat"=w635, "Input"=w636) -> (w587:T7)
            n142 = Bundle By Name(cluster=T7 {"CID"="", "Comm Stat"=FALSE, "Input"=[]} ("constatnt"), "CID"=w565, "Comm Stat"=w634, "Input"=w633) -> (w583:T7)
            n143 = Bundle By Name(cluster=T7 {"CID"="", "Comm Stat"=FALSE, "Input"=[]} ("constatnt"), "CID"=w564, "Comm Stat"=w625, "Input"=w626) -> (w579:T7)
            n144 = Bundle By Name(cluster=T7 {"CID"="", "Comm Stat"=FALSE, "Input"=[]} ("constatnt"), "CID"=w563, "Comm Stat"=w624, "Input"=w623) -> (w574:T7)
            n145 = Bundle By Name(cluster=T7 {"CID"="", "Comm Stat"=FALSE, "Input"=[]} ("constatnt"), "CID"=w562, "Comm Stat"=w615, "Input"=w616) -> (w570:T7)
            n146 = call "AB_PLC_testing.vi"("error in (no error)"=w558) -> ("AB plc output 10"=w553:T7, "AB plc output 9"=w554:T7, "AB plc output 8"=w555:T7, "AB plc output 7"=w556:T7, "error in (no error) 2"=w557:errorcluster)  [unwired: 6 in]
            n147 = Build Array(w556, w555, w554, w553) -> (w552:T10)
            n148 = case shown="Error" w598 {
              tunnel: w599 -> [w677 _]
              tunnel: [w677 w679] -> w596
              tunnel: w597 -> [_ w680]
              frame No Error {
              }
              frame Error {
                n149 = Bundle By Name(cluster=w680, "Comm Stat"=FALSE) -> (w679:T7)
              }
            }
            n150 = case shown="Error" w585 {
              tunnel: w587 -> [w668 _]
              tunnel: [w668 w670] -> w584
              tunnel: w586 -> [_ w671]
              frame No Error {
              }
              frame Error {
                n151 = Bundle By Name(cluster=w671, "Comm Stat"=FALSE) -> (w670:T7)
              }
            }
            n152 = case shown="Error" w580 {
              tunnel: w583 -> [w664 _]
              tunnel: [w664 w666] -> w581
              tunnel: w582 -> [_ w667]
              frame No Error {
              }
              frame Error {
                n153 = Bundle By Name(cluster=w667, "Comm Stat"=FALSE) -> (w666:T7)
              }
            }
            n154 = case shown="Error" w577 {
              tunnel: w579 -> [w660 _]
              tunnel: [w660 w662] -> w576
              tunnel: w578 -> [_ w663]
              frame No Error {
              }
              frame Error {
                n155 = Bundle By Name(cluster=w663, "Comm Stat"=FALSE) -> (w662:T7)
              }
            }
            n156 = case shown="Error" w575 {
              tunnel: w574 -> [w656 _]
              tunnel: [w656 w658] -> w572
              tunnel: w573 -> [_ w659]
              frame No Error {
              }
              frame Error {
                n157 = Bundle By Name(cluster=w659, "Comm Stat"=FALSE) -> (w658:T7)
              }
            }
            n158 = case shown="No Error" w571 {
              tunnel: w570 -> [w652 _]
              tunnel: [w652 w654] -> w568
              tunnel: w569 -> [_ w655]
              frame No Error {
              }
              frame Error {
                n159 = Bundle By Name(cluster=w655, "Comm Stat"=FALSE) -> (w654:T7)
              }
            }
            n160 = Build Array (concatenate)(w596, w584, w581, w576, w572, w568, w552) -> (w595:T10)
            n161 = for {
              tunnel: w595 -> [w672] mode=indexing
              tunnel: w649 -> [w676]
              tunnel: [w675] -> w648
              tunnel: w647 -> [w674]
              tunnel: [w673] -> w646
              n162 = Enqueue Element(queue=w676, element=w672, error in (no error)=w674) -> (queue out=w675:refnum<queue>, error out=w673:errorcluster)  [unwired: 1 in, 1 out]
            }
          }
          event "stop": Value Change {
            n163 = event-data() -> ()  [unwired: 1 in, 1 out]
            n164 = call "Login to stop exe.vi"("error in (no error) 2"=w682) -> ("error in (no error)"=w681:errorcluster, "Success"=w683:bool)  [unwired: 7 in]
          }
        }
        "Stop from Main" <- w467
        n165 = case shown="True" w417 {
          selector: w417 -> [w512 _]
          tunnel: [w511 FALSE] -> w423
          tunnel: w422 -> [w513 w515]
          frame False {
            n166 = Select(t=w512, s=w513, f=TRUE) -> (s? t:f=w511:bool)
          }
          frame True {
            n167 = call "ErrorLogVI.vi"("Error In"=w515, "Station"=" ST 1 ") -> ()  [unwired: 10 in]
          }
        }
        n168 = case shown="True" w432 {
          selector: w432 -> [w547 _]
          tunnel: [w546 FALSE] -> w434
          tunnel: w433 -> [w548 w550]
          frame False {
            n169 = Select(t=w547, s=w548, f=TRUE) -> (s? t:f=w546:bool)
          }
          frame True {
            n170 = call "ErrorLogVI.vi"("Error In"=w550, "Station"=" ST 2 ") -> ()  [unwired: 10 in]
          }
        }
        n171 = case shown="True" w418 {
          selector: w418 -> [w540 _]
          tunnel: [w539 FALSE] -> w431
          tunnel: w428 -> [w541 w543]
          frame False {
            n172 = Select(t=w540, s=w541, f=TRUE) -> (s? t:f=w539:bool)
          }
          frame True {
            n173 = call "ErrorLogVI.vi"("Error In"=w543, "Station"=" ST 3 ") -> ()  [unwired: 10 in]
          }
        }
        n174 = case shown="True" w419 {
          selector: w419 -> [w533 _]
          tunnel: [w532 FALSE] -> w430
          tunnel: w429 -> [w534 w536]
          frame False {
            n175 = Select(t=w533, s=w534, f=TRUE) -> (s? t:f=w532:bool)
          }
          frame True {
            n176 = call "ErrorLogVI.vi"("Error In"=w536, "Station"=" ST 4 ") -> ()  [unwired: 10 in]
          }
        }
        n177 = case shown="True" w420 {
          selector: w420 -> [w526 _]
          tunnel: [w525 FALSE] -> w427
          tunnel: w426 -> [w527 w529]
          frame False {
            n178 = Select(t=w526, s=w527, f=TRUE) -> (s? t:f=w525:bool)
          }
          frame True {
            n179 = call "ErrorLogVI.vi"("Error In"=w529, "Station"=" ST 5 ") -> ()  [unwired: 10 in]
          }
        }
        n180 = case shown="True" w421 {
          selector: w421 -> [w519 _]
          tunnel: [w518 FALSE] -> w425
          tunnel: w424 -> [w520 w522]
          frame False {
            n181 = Select(t=w519, s=w520, f=TRUE) -> (s? t:f=w518:bool)
          }
          frame True {
            n182 = call "ErrorLogVI.vi"("Error In"=w522, "Station"=" ST 6 ") -> ()  [unwired: 10 in]
          }
        }
      }
      n183 = call <vilib>:"Clear Errors.vi"("error in (no error)"=w115) -> ("error out"=w114:errorcluster)  [unwired: 5 in, 1 out]
      n184 = call <vilib>:"Clear Errors.vi"("error in (no error)"=w77) -> ("error out"=w93:errorcluster)  [unwired: 5 in, 1 out]
      n185 = call <vilib>:"Clear Errors.vi"("error in (no error)"=w69) -> ("error out"=w91:errorcluster)  [unwired: 5 in, 1 out]
      n186 = call <vilib>:"Clear Errors.vi"("error in (no error)"=w112) -> ("error out"=w117:errorcluster)  [unwired: 5 in, 1 out]
      n187 = call <vilib>:"Clear Errors.vi"("error in (no error)"=w76) -> ("error out"=w92:errorcluster)  [unwired: 5 in, 1 out]
      n188 = call <vilib>:"Clear Errors.vi"("error in (no error)"=w70) -> ("error out"=w90:errorcluster)  [unwired: 5 in, 1 out]
      n189 = call <vilib>:"Clear Errors.vi"("error in (no error)"=w71) -> ("error out"=w89:errorcluster)  [unwired: 5 in, 1 out]
      n190 = call-dynamic "Shutdown.vi"("error in"=w93, "Modbus master in"=w84) -> ("error out"=w78:errorcluster)  [unwired: 9 in]
      n191 = call-dynamic "Shutdown.vi"("error in"=w91, "Modbus master in"=w86) -> ("error out"=w74:errorcluster)  [unwired: 9 in]
      n192 = Flush Queue(queue=w136, error in (no error)=w114) -> (queue out=w137:refnum<queue>, error out=w138:errorcluster)  [unwired: 1 out]
      n193 = call-dynamic "Shutdown.vi"("error in"=w117, "Modbus master in"=w116) -> ("error out"=w79:errorcluster)  [unwired: 9 in]
      n194 = call-dynamic "Shutdown.vi"("error in"=w92, "Modbus master in"=w85) -> ("error out"=w75:errorcluster)  [unwired: 9 in]
      n195 = call-dynamic "Shutdown.vi"("error in"=w90, "Modbus master in"=w87) -> ("error out"=w73:errorcluster)  [unwired: 9 in]
      n196 = call-dynamic "Shutdown.vi"("error in"=w89, "Modbus master in"=w88) -> ("error out"=w72:errorcluster)  [unwired: 9 in]
      n197 = flat-sequence {
        tunnel: w123 -> [w158]
        tunnel: [w158] -> w81
        frame #0 {
          n198 = Wait (ms)(milliseconds to wait=u32 1000) -> ()  [unwired: 1 out]
        }
      }
      n199 = call <vilib>:"Clear Errors.vi"("error in (no error)"=w66) -> ("error out"=w65:errorcluster)  [unwired: 5 in, 1 out]
      n200 = Release Queue(queue=w137, error in (no error)=w138) -> (error out=w80:errorcluster)  [unwired: 1 in, 2 out]
      n201 = call <vilib>:"DB Tools Close Connection.vi"("error in (no error)"=w65, "connection reference"=w67) -> ("error out"=w120:errorcluster)  [unwired: 5 in]
      n202 = Unbundle By Name(w120) -> ()  [unwired: 1 out]
      n203 = Merge Errors(w112, w77, w76, w69, w70, w71, w79, w78, w75, w74, w73, w72, w81, w80) -> (w113:errorcluster)
    }
  }
  n204 = call <vilib>:"Clear Errors.vi"("error in (no error)"=w3) -> ("error out"=w5:errorcluster)  [unwired: 5 in, 1 out]
  n205 = call "ErrorLogVI.vi"("Error In"=w3, "Station"="") -> ()  [unwired: 10 in]
  n206 = property class="App"(error in=w5) -> (error out=w8:errorcluster, "App.Kind"=w7:T11)  [unwired: 1 in, 1 out]
  n207 = case shown="\"Run Time System\"" w7 {
    tunnel: [w703 w706] -> w4
    tunnel: w8 -> [w704 w706]
    frame "Run Time System" {
      n208 = control-ref of="This VI"() -> (w705:refnum<vi>)
      n209 = invoke class="VI" method="FP.Close"(reference=w705, error in=w704) -> (error out=w703:errorcluster)  [unwired: 1 in, 2 out]
    }
    frame "Development System", Default {
    }
  }
  n210 = Unbundle By Name(w4) -> ()  [unwired: 1 out]
